vi "Facade.vi"(0 "Data In":T4, 2 "Display State In":T2, 3 "Container State":T3) -> (6 "Data Out":T4, 7 "Display State Out":T2, 8 "Action":T1)   [LabVIEW 2020, in "Advanced Options (G3).xctl"]
uses:
  Advanced Options (G3).xctl
  Advanced Options (G3).ctl
  <vilib>/_xctls/Container State.ctl
  State.ctl
  <vilib>/_xctls/Action.ctl
  <vilib>/_xctls/XControlSupport.lvlib
panel:
  in  "Alternate polarity":bool
  in  "Expression":string
  in  "Variable":u16(ring)
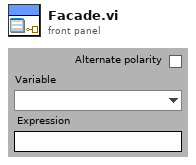
[diagram p1: front panel]
types:
  T1 = typedef "XControlSupport.lvlib/Action.ctl" = cluster{"Data Changed?":bool, "State Changed?":bool, "Action Name":string}
  T2 = typedef "Advanced Options (G3).xctl/State.ctl" = cluster{"VarNames":string[], "show vars":bool}
  T3 = typedef "XControlSupport.lvlib/Container State.ctl" = cluster{"Indicator?":bool, "Run Mode?":bool, " Refnum":refnum<vi>}
  T4 = typedef "Advanced Options (G3).xctl/Advanced Options (G3).ctl" = cluster{"AltPol":bool, "Var":string, "Expr":string}
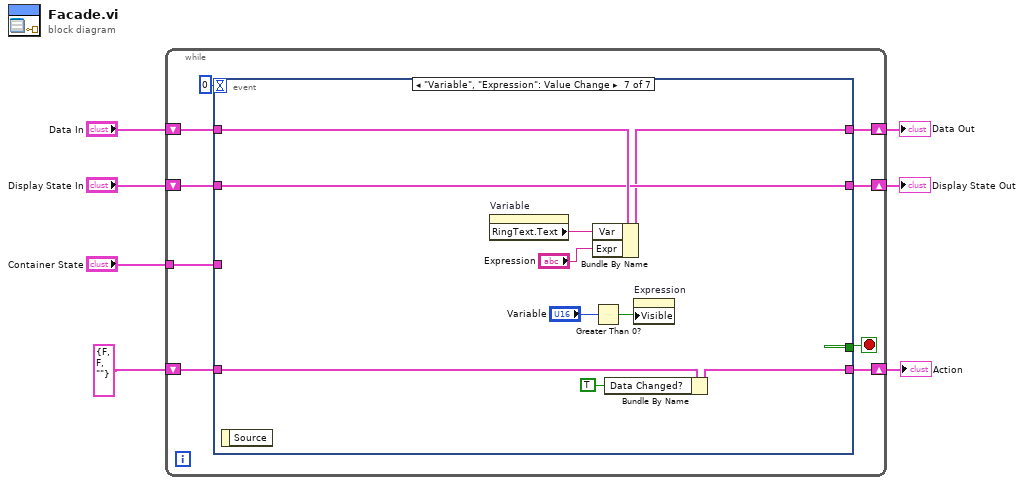
[diagram p0: block diagram]
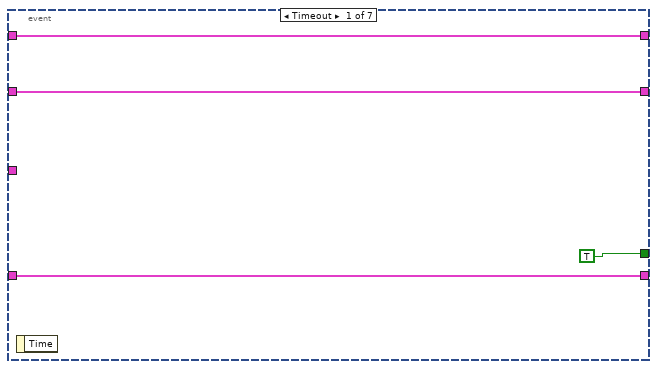
[diagram p2: hidden frame]
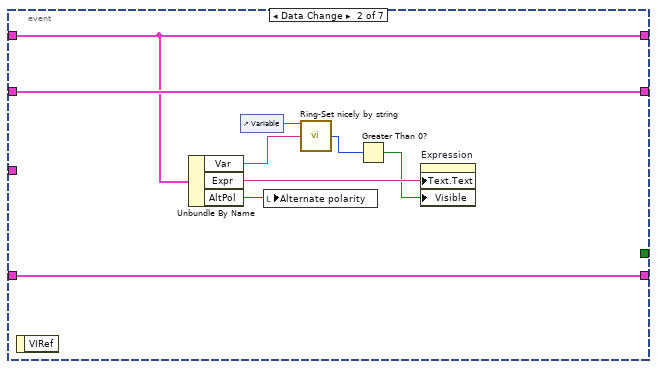
[diagram p3: hidden frame]
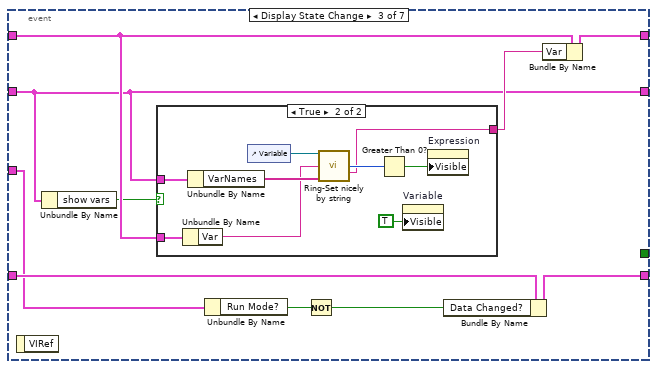
[diagram p4: hidden frame]
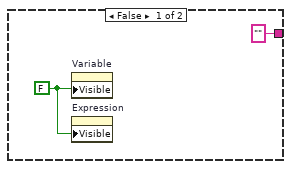
[diagram p5: hidden frame]
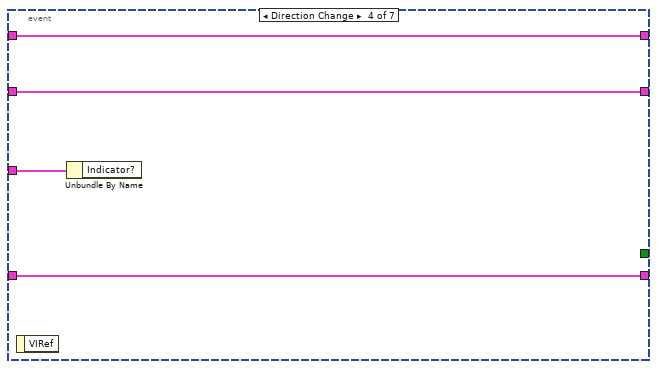
[diagram p6: hidden frame]
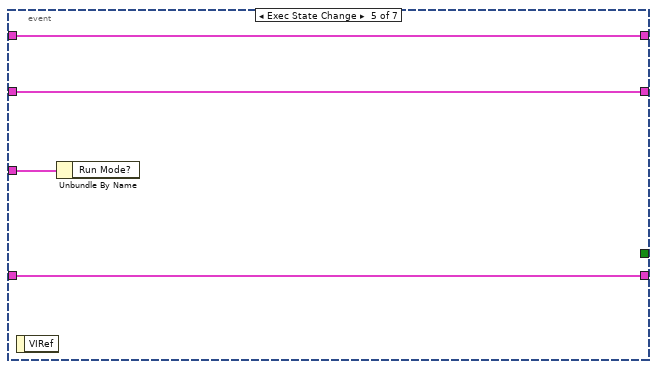
[diagram p7: hidden frame]
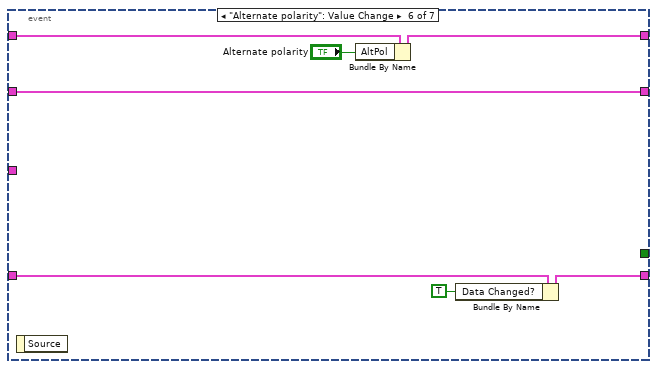
[diagram p8: hidden frame]
diagram:
  n1 = while {
    shift-right: [w15] -> w4
    shift-left: "Display State In" -> [w16]
    tunnel: "Container State" -> [w12]
    shift-right: [w10] -> w7
    shift-left: "Data In" -> [w11]
    shift-right: [w8] -> w2
    shift-left: T1 {"Data Changed?"=FALSE, "State Changed?"=FALSE, "Action Name"=""} ("Action") -> [w9]
    stop <- w14 stop-if-true
    n2 = event shown="[6] \"Variable\", \"Expression\": Value Change" {
      selector: _ -> [_ _ _ _ _ _ _]
      dyn-events: _ -> [_ _ _ _ _ _ _]
      timeout: 0 -> [_ _ _ _ _ _ _]
      tunnel: w16 -> [w18 w29 w34 w53 w57 w64 w74]
      tunnel: [w18 w29 w34 w53 w57 w64 w74] -> w15
      tunnel: [TRUE _ _ _ _ _ _] -> w14
      tunnel: w12 -> [_ _ w32 w54 w58 _ _]
      tunnel: w11 -> [w17 w26 w38 w52 w56 w65 w75]
      tunnel: [w17 w26 w37 w52 w56 w62 w72] -> w10
      tunnel: [w19 w28 w35 w51 w55 w60 w71] -> w8
      tunnel: w9 -> [w19 w28 w39 w51 w55 w63 w73]
      event Timeout {
        n3 = event-data() -> ()  [unwired: 1 in, 1 out]
      }
      event Data Change {
        n4 = event-data() -> ()  [unwired: 1 in, 1 out]
        n5 = Unbundle By Name(w26) -> ("Var"=w25:string, "Expr"=w23:string, "AltPol"=w21:bool)
        n6 = control-ref of="Variable"() -> (w27:refnum<vi>)
        n7 = local write "Alternate polarity"(w21) -> ()
        n8 = call "Ring-Set nicely by string.vi"("Ring in"=w27, "Device"=w25) -> ("Index"=w24:i32)  [unwired: 10 in, 3 out]
        n9 = Greater Than 0?(x=w24) -> (x > 0?=w22:bool)
        n10 = property on="Expression" class="Str"("Text.Text"=w23, "Visible"=w22) -> ()  [unwired: 2 in, 2 out]
      }
      event Display State Change {
        n11 = event-data() -> ()  [unwired: 1 in, 1 out]
        n12 = Unbundle By Name(w34) -> ("show vars"=w33:bool)
        n13 = case shown="True" w33 {
          tunnel: w34 -> [_ w50]
          tunnel: w38 -> [_ w49]
          tunnel: ["" ("Selection") w43] -> w36
          frame False {
            w40 = FALSE
            n14 = property on="Variable" class="Ring (strict)"("Visible"=w40) -> ()  [unwired: 2 in, 2 out]
            n15 = property on="Expression" class="Str"("Visible"=w40) -> ()  [unwired: 2 in, 2 out]
          }
          frame True {
            n16 = Unbundle By Name(w49) -> ("Var"=w46:string)
            n17 = Unbundle By Name(w50) -> ("VarNames"=w47:string[])
            n18 = control-ref of="Variable"() -> (w48:refnum<vi>)
            n19 = call "Ring-Set nicely by string.vi"("Ring in"=w48, "Device"=w46, "Strings []"=w47) -> ("Index"=w44:i32, "Selection"=w43:string)  [unwired: 9 in, 2 out]
            n20 = Greater Than 0?(x=w44) -> (x > 0?=w45:bool)
            n21 = property on="Variable" class="Ring (strict)"("Visible"=TRUE) -> ()  [unwired: 2 in, 2 out]
            n22 = property on="Expression" class="Str"("Visible"=w45) -> ()  [unwired: 2 in, 2 out]
          }
        }
        n23 = Unbundle By Name(w32) -> ("Run Mode?"=w31:bool)
        n24 = Not(x=w31) -> (.not. x?=w30:bool)
        n25 = Bundle By Name(cluster=w39, "Data Changed?"=w30) -> (w35:T1)
        n26 = Bundle By Name(cluster=w38, "Var"=w36) -> (w37:T4)
      }
      event Direction Change {
        n27 = event-data() -> ()  [unwired: 1 in, 1 out]
        n28 = Unbundle By Name(w54) -> ()  [unwired: 1 out]
      }
      event Exec State Change {
        n29 = event-data() -> ()  [unwired: 1 in, 1 out]
        n30 = Unbundle By Name(w58) -> ()  [unwired: 1 out]
      }
      event "Alternate polarity": Value Change {
        n31 = event-data() -> ()  [unwired: 1 in, 1 out]
        n32 = Bundle By Name(cluster=w65, "AltPol"="Alternate polarity") -> (w62:T4)
        n33 = Bundle By Name(cluster=w63, "Data Changed?"=TRUE) -> (w60:T1)
      }
      event "Variable", "Expression": Value Change {
        n34 = event-data() -> ()  [unwired: 1 in, 1 out]
        n35 = property on="Variable" class="Ring (strict)"() -> ("RingText.Text"=w69:string)  [unwired: 2 in, 2 out]
        n36 = Bundle By Name(cluster=w75, "Var"=w69, "Expr"="Expression") -> (w72:T4)
        n37 = Greater Than 0?(x="Variable") -> (x > 0?=w67:bool)
        n38 = Bundle By Name(cluster=w73, "Data Changed?"=TRUE) -> (w71:T1)
        n39 = property on="Expression" class="Str"("Visible"=w67) -> ()  [unwired: 2 in, 2 out]
      }
    }
  }
  "Display State Out" <- w4
  "Data Out" <- w7
  "Action" <- w2
